vi "Word_Set_Chart_Colors.vi"(0 "Word.InlineShapes":refnum<k7>, 1 "MarkerStyle":i32(ring)=-4105 items=["xlMarkerStyleAutomatic"=-4105, "xlMarkerStyleCircle"=8, "xlMarkerStyleDash"=-4115, "xlMarkerStyleDiamond"=2, "xlMarkerStyleDot"=-4118, "xlMarkerStyleNone"=-4142, "xlMarkerStylePicture"=-4147, "xlMarkerStylePlus"=9, "xlMarkerStyleSquare"=1, "xlMarkerStyleStar"=5, "xlMarkerStyleTriangle"=3, "xlMarkerStyleX"=-4168], 2 "weight":i16, 9 "chart index":u16, 11 "error in":errorcluster, 12 "plot colors":u32[](array[colorbox]), 13 "plot area color":u32(colorbox), 14 "chart area color":u32(colorbox)) -> (15 "error out":errorcluster)   [LabVIEW 2010, in "NI_ReportGenerationToolkit.lvlib"]
uses:
  <vilib>/addons/_office/NI_ReportGenerationToolkit.lvlib
panel:
  in  "Graph.Series":refnum<k7>
  in  "Graph.Chart":refnum<k7>
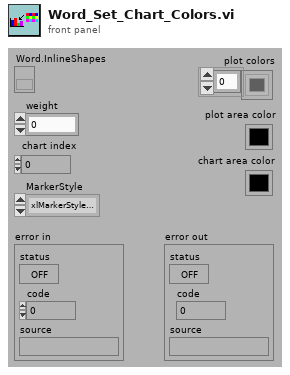
[diagram p1: front panel]
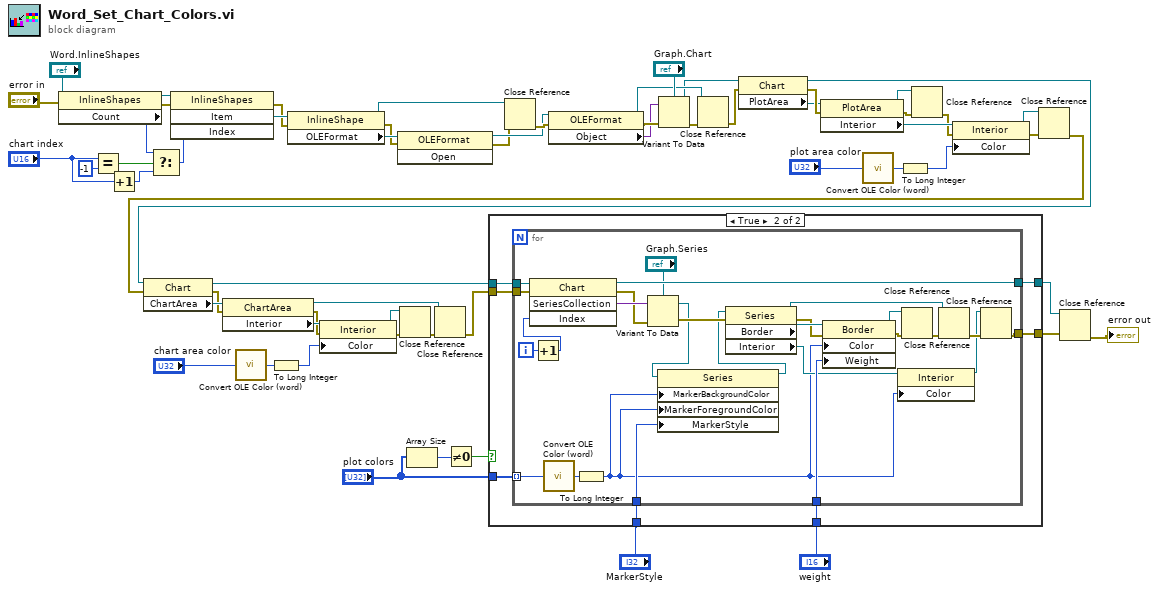
[diagram p0: block diagram]
diagram:
  n1 = property class="InlineShapes"(reference="Word.InlineShapes", error in="error in") -> (reference out=w47:refnum<k7>, error out=w58:errorcluster, "Count"=w38:i32)
  n2 = Equal?(x="chart index", y=i16 -1) -> (x = y?=w42:bool)
  n3 = Increment(x="chart index") -> (x+1=w40:u16)
  n4 = Select(t=w38, s=w42, f=w40) -> (s? t:f=w37:i32)
  n5 = invoke class="InlineShapes" method="Item"(reference=w47, error in=w58, "Index"=w37) -> (error out=w49:errorcluster, "Item"=w50:refnum<k7>)  [unwired: 1 in, 2 out]
  n6 = call <vilib>:"Convert OLE Color (word).vi"("color in"="chart area color") -> ("color out"=w20:u32)
  n7 = To Long Integer(number=w20) -> (32bit integer=w10:i32)
  n8 = property class="InlineShape"(reference=w50, error in=w49) -> (reference out=w53:refnum<k7>, error out=w8:errorcluster, "OLEFormat"=w9:refnum<k7>)
  n9 = invoke class="OLEFormat" method="Open"(reference=w9, error in=w8) -> (reference out=w7:refnum<k7>, error out=w6:errorcluster)  [unwired: 1 in, 1 out]
  n10 = Array Size(array="plot colors") -> (size(s)=w2:i32)
  n11 = Not Equal To 0?(x=w2) -> (x != 0?=w27:bool)
  n12 = Close Reference(reference=w53, error in (no error)=w6) -> (error out=w52:errorcluster)
  n13 = property class="OLEFormat"(reference=w7, error in=w52) -> (reference out=w51:refnum<k7>, error out=w57:errorcluster, "Object"=w56:variant)
  n14 = Variant To Data(error in=w57, Variant=w56, type="Graph.Chart") -> (error out=w54:errorcluster, data=w36:refnum<k7>)
  n15 = Close Reference(reference=w51, error in (no error)=w54) -> (error out=w46:errorcluster)
  n16 = property class="Chart"(reference=w36, error in=w46) -> (reference out=w22:refnum<k7>, error out=w44:errorcluster, "PlotArea"=w26:refnum<k7>)
  n17 = property class="PlotArea"(reference=w26, error in=w44) -> (reference out=w32:refnum<k7>, error out=w33:errorcluster, "Interior"=w31:refnum<k7>)
  n18 = call <vilib>:"Convert OLE Color (word).vi"("color in"="plot area color") -> ("color out"=w43:u32)
  n19 = To Long Integer(number=w43) -> (32bit integer=w11:i32)
  n20 = Close Reference(reference=w32, error in (no error)=w33) -> (error out=w30:errorcluster)
  n21 = property class="Interior"(reference=w31, error in=w30, "Color"=w11) -> (reference out=w28:refnum<k7>, error out=w29:errorcluster)
  n22 = Close Reference(reference=w28, error in (no error)=w29) -> (error out=w21:errorcluster)
  n23 = property class="Chart"(reference=w22, error in=w21) -> (reference out=w23:refnum<k7>, error out=w16:errorcluster, "ChartArea"=w25:refnum<k7>)
  n24 = property class="ChartArea"(reference=w25, error in=w16) -> (reference out=w13:refnum<k7>, error out=w15:errorcluster, "Interior"=w24:refnum<k7>)
  n25 = property class="Interior"(reference=w24, error in=w15, "Color"=w10) -> (reference out=w14:refnum<k7>, error out=w17:errorcluster)
  n26 = Close Reference(reference=w14, error in (no error)=w17) -> (error out=w18:errorcluster)
  n27 = Close Reference(reference=w13, error in (no error)=w18) -> (error out=w12:errorcluster)
  n28 = case shown="True" w27 {
    tunnel: "MarkerStyle" -> [_ w68]
    tunnel: "weight" -> [_ w67]
    tunnel: [w60 w66] -> w5
    tunnel: [w61 w65] -> w4
    tunnel: w23 -> [w61 w64]
    tunnel: w12 -> [w60 w63]
    tunnel: "plot colors" -> [_ w62]
    frame False {
    }
    frame True {
      n29 = for {
        tunnel: w68 -> [w94]
        tunnel: w67 -> [w93]
        tunnel: [w92] -> w66
        tunnel: [w91] -> w65
        tunnel: w64 -> [w90]
        tunnel: w63 -> [w89]
        tunnel: w62 -> [w69] mode=indexing
        i -> [w71]
        n30 = Increment(x=w71) -> (x+1=w70:i32)
        n31 = invoke class="Chart" method="SeriesCollection"(reference=w90, error in=w89, "Index"=w70) -> (reference out=w91:refnum<k7>, error out=w86:errorcluster, "SeriesCollection"=w87:variant)  [unwired: 1 in, 1 out]
        n32 = call <vilib>:"Convert OLE Color (word).vi"("color in"=w69) -> ("color out"=w76:u32)
        n33 = To Long Integer(number=w76) -> (32bit integer=w72:i32)
        n34 = Variant To Data(error in=w86, Variant=w87, type="Graph.Series") -> (error out=w85:errorcluster, data=w79:refnum<k7>)
        n35 = property class="Series"(reference=w79, "MarkerBackgroundColor"=w72, "MarkerForegroundColor"=w72, "MarkerStyle"=w94) -> (reference out=w78:refnum<k7>)  [unwired: 1 in, 1 out]
        n36 = property class="Series"(reference=w78, error in=w85) -> (reference out=w80:refnum<k7>, error out=w84:errorcluster, "Border"=w88:refnum<k7>, "Interior"=w77:refnum<k7>)
        n37 = property class="Border"(reference=w88, error in=w84, "Color"=w72, "Weight"=w93) -> (reference out=w81:refnum<k7>, error out=w82:errorcluster)
        n38 = property class="Interior"(reference=w77, "Color"=w72) -> (reference out=w74:refnum<k7>)  [unwired: 1 in, 1 out]
        n39 = Close Reference(reference=w81, error in (no error)=w82) -> (error out=w83:errorcluster)
        n40 = Close Reference(reference=w80, error in (no error)=w83) -> (error out=w75:errorcluster)
        n41 = Close Reference(reference=w74, error in (no error)=w75) -> (error out=w92:errorcluster)
      }
    }
  }
  n42 = Close Reference(reference=w4, error in (no error)=w5) -> (error out=→"error out":errorcluster)
